vi "AvaSpec Control.vi"(8 "error in (no error)":errorcluster, 9 "Sphere Indicator":T1, 10 "Master":refnum<queue>, 11 "Subpanel ref":refnum<vi>) -> (0 "error out":errorcluster)   [LabVIEW 2014, in "Instrument Launcher.lvlib"]
uses:
  Support/MeasurementControl Message Queue Folder/Message Cluster.ctl
  avantesSpectrometer/Acquisition/Sphere Indicator.ctl
  avantesSpectrometer/Settings/Measurement Type.ctl
  Instrument Launcher.lvlib
  avantesSpectrometer/Acquisition/AvaSpec Acquisition.lvlib
  Support/MeasurementControl Message Queue Folder/MeasurementControl Message Queue.lvlib
  avantesSpectrometer/AvaSpec.lvlib
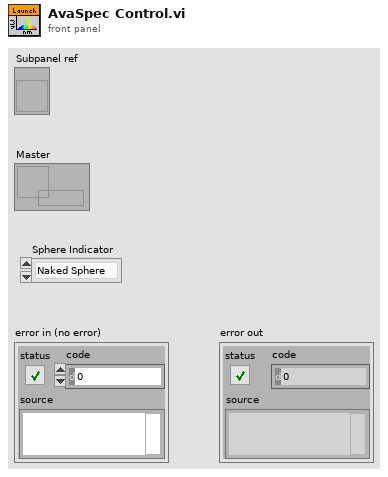
[diagram p1: front panel]
types:
  T1 = typedef "AvaSpec.lvlib/Sphere Indicator.ctl" = enum16{"Naked Sphere", "Insulated Sphere"}
  T2 = typedef "AvaSpec.lvlib/AvaSpec Acquisition.lvlib/Measurement Type.ctl" = enum16{"Normal", "Calibration", "Dark"}
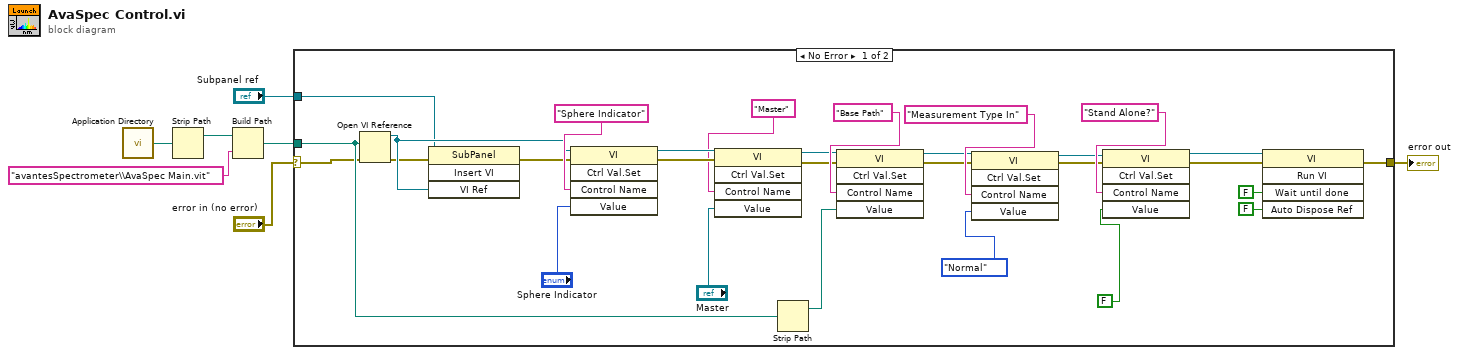
[diagram p0: block diagram]
diagram:
  n1 = call <vilib>:"Application Directory.vi"() -> ("Application Directory"=w2:path)
  n2 = Strip Path(path=w2) -> (stripped path=w3:path)  [unwired: 1 out]
  n3 = Build Path(base path=w3, name or relative path="avantesSpectrometer\\AvaSpec Main.vit") -> (appended path=w1:path)
  n4 = case shown="No Error" "error in (no error)" {
    selector: "error in (no error)" -> [w8 w37]
    tunnel: w1 -> [w12 _]
    tunnel: "Subpanel ref" -> [w15 _]
    tunnel: [w14 w37] -> w6
    frame No Error {
      n5 = Open VI Reference(vi path=w12, error in (no error)=w8) -> (vi reference=w18:refnum<vi>, error out=w16:errorcluster)  [unwired: 4 in]
      n6 = invoke on="Invoke Node" class="SubPanel" method="Insert VI"(reference=w15, error in=w16, "VI Ref"=w18) -> (error out=w17:errorcluster)  [unwired: 1 in, 3 out]
      n7 = invoke class="VI" method="Ctrl Val.Set"(reference=w18, error in=w17, "Control Name"="Sphere Indicator", "Value"="Sphere Indicator") -> (reference out=w34:refnum<vi>, error out=w35:errorcluster)  [unwired: 1 in, 3 out]
      n8 = invoke class="VI" method="Ctrl Val.Set"(reference=w34, error in=w35, "Control Name"="Master", "Value"="Master") -> (reference out=w10:refnum<vi>, error out=w9:errorcluster)  [unwired: 1 in, 3 out]
      n9 = Strip Path(path=w12) -> (stripped path=w11:path)  [unwired: 1 out]
      n10 = invoke class="VI" method="Ctrl Val.Set"(reference=w10, error in=w9, "Control Name"="Base Path", "Value"=w11) -> (reference out=w23:refnum<vi>, error out=w22:errorcluster)  [unwired: 1 in, 3 out]
      n11 = invoke class="VI" method="Ctrl Val.Set"(reference=w23, error in=w22, "Control Name"="Measurement Type In", "Value"=Measurement_Type."Normal" ("Measurement Type In")) -> (reference out=w21:refnum<vi>, error out=w20:errorcluster)  [unwired: 1 in, 3 out]
      n12 = invoke class="VI" method="Ctrl Val.Set"(reference=w21, error in=w20, "Control Name"="Stand Alone?", "Value"=FALSE) -> (reference out=w27:refnum<vi>, error out=w28:errorcluster)  [unwired: 1 in, 3 out]
      n13 = invoke class="VI" method="Run VI"(reference=w27, error in=w28, "Wait until done"=FALSE ("Wait Until Done"), "Auto Dispose Ref"=FALSE ("Auto Dispose Reference")) -> (error out=w14:errorcluster)  [unwired: 1 in, 4 out]
    }
    frame Error {
    }
  }
  "error out" <- w6
